vi "observacao.vi"() -> ()   [LabVIEW 2012] (continued)
                    n664 = global write "Global_Telescopio.vi" "T cup"(w581) -> ()
                    "Dome on Target" <- TRUE
                  }
                  frame True {
                    # "Abrir Trapeira"
                    n665 = case shown="False" w585 {
                      tunnel: [7 w590] -> w584
                      frame False {
                        w589 = u16 4 items=["ZERO", "AH", "DEC", "TUBO", "CUP"] ("Controlador")
                        # "Aguardar abertura Trap."
                        # "CLP Pronto"
                        n666 = call "Monta Comando.vi"("Comando"="ABRIR", "Dispositivo"="TRAPEIRA" ("Comando"), "Controlador"=w589) -> ()  [unwired: 4 in, 3 out]
                      }
                      frame True {
                        # "CLP Busy"
                        n667 = local read "TimeoutCUP"() -> (w592:u32)
                        n668 = call "TickTimeout.vi"("msInicial"=w592, "msTimeout"=u32 5000) -> ("Timeout"=w591:bool)  [unwired: 2 out]
                        n669 = case shown="True" w591 {
                          tunnel: [6 3] -> w590
                          frame False {
                          }
                          frame True {
                          }
                        }
                      }
                    }
                  }
                }
              }
              frame 7 {
                w596 = u16 6 items=["Alarme", "Atencao", "Erro", "Ocupado", "TBD", "LCB", "Trapeira", "Paravento", "DomoRap", "DomoCW", "DomoCCW", "TBD", "Em movimento", "TBD"] ("NomeStatus")
                # "Aqui também caberia um Timeout?"
                # "Aguarda abertura Trapeira"
                # "Também poderia ser testado o bit \"Em movimento\".\nNeste caso o código do \"IF\" deve ser permutado."
                n670 = call "Bit Status CUP.vi"("NomeStatus"=w596) -> ("StatBit"=w597:bool)
                n671 = case shown="True" w597 {
                  tunnel: [7 0] -> w598
                  frame False {
                    # "Ainda movendo...\nAGUARDAR"
                  }
                  frame True {
                    w601 = TRUE ("Dome on Target")
                    # "Trapeira aberta.\nFIM"
                    n672 = call "TickTimeout.vi"() -> ("msTick"=w600:u32)  [unwired: 2 in, 2 out]
                    n673 = local write "Dome on Target"(w601) -> ()
                    n674 = local write "RefreshShutterState"(w601) -> ()
                    n675 = local write "TimeoutCUP"(w600) -> ()
                    n676 = global write "Global_Telescopio.vi" "T cup"(w600) -> ()
                  }
                }
              }
            }
            n677 = case shown="True" w460 {
              tunnel: w449 -> [w480 _]
              tunnel: [w479 "POINT" ("Boolean Text.Text")] -> w448
              frame False {
                n678 = case shown="True" w480 {
                  tunnel: ["POINT" ("Boolean Text.Text") "STOP" ("Boolean Text.Text")] -> w479
                  frame False {
                  }
                  frame True {
                  }
                }
              }
              frame True {
                w483 = TRUE
                # "MUDANÇA:\n22/6/2011 \nHab. Guider"
                n679 = local read "ChkDomeEnable"() -> (w484:bool)
                n680 = global write "Global_Telescopio.vi" "Botão GO = STOP"(FALSE) -> ()
                n681 = local write "LED GUIDER"(w483) -> ()
                n682 = local write "GUIDER"(w483) -> ()
                n683 = local write "DOME"(w484) -> ()
              }
            }
            n684 = Tick Count (ms)() -> (millisecond timer value=w441:u32)
            n685 = Subtract(x=w441, y=w447) -> (x-y=w440:u32)
            n686 = Less?(x=w440, y=w442) -> (x < y?=w443:bool)
            n687 = control-ref of="BtTargetPoint"() -> (w477:refnum<vi>)
            n688 = case shown="True" w443 {
              tunnel: w442 -> [_ w478]
              frame False {
              }
              frame True {
                n689 = Wait Until Next ms Multiple(millisecond multiple=w478) -> ()  [unwired: 1 out]
              }
            }
            n690 = property class="Bool"(reference=w477, "Boolean Text.Text"=w448) -> ()  [unwired: 1 in, 2 out]
            n691 = call "PROTECAO.vi"("Estado In"=w453) -> ("Estado Out"=w452:i32)  [unwired: 2 in]
            n692 = local write "statCUP"(w452) -> ()
            "statCUP 2" <- "statCUP"
            "Erro Lim" <- 15 ("y")
            "Erro PROTEC" <- 10 ("y")
          }
          frame #4 {
            # "CHECA FINAL DO APONTAMENTO"
            # "ascensão reta = tempo sideral - ângulo horário (2)"
            n693 = local read "LedPointing"() -> (w899:bool)
            n694 = case shown="True" w899 {
              frame False {
                n695 = property on="DOME" class="Bool (strict)"("Disabled"=u8 0) -> ()  [unwired: 2 in, 2 out]
              }
              frame True {
                n696 = local read "statCUP"() -> (w904:i32)
                n697 = local read "statAH"() -> (w903:i32)
                n698 = local read "statDEC"() -> (w905:i32)
                n699 = Compound Arithmetic op=ADD(w904, w903, w905) -> (w906:i32)
                n700 = Greater Than 0?(x=w906) -> (x > 0?=w902:bool)
                n701 = case shown="False" w902 {
                  selector: w902 -> [w907 _]
                  frame False {
                    w910 = TRUE
                    n702 = local read "ChkPointPrecessed"() -> (w908:bool)
                    n703 = local read "StrPointObjName"() -> (w913:string)
                    n704 = local read "StrPointObjRA"() -> (w912:string)
                    n705 = local read "StrPointObjDEC"() -> (w911:string)
                    n706 = local write "LedPointing"(w907) -> ()
                    n707 = property on="LedPointing" class="Bool (strict)"("Visible"=w907) -> ()  [unwired: 2 in, 2 out]
                    n708 = case shown="True" w908 {
                      tunnel: ["2000.0" ("Saída") w915] -> w909
                      frame False {
                      }
                      frame True {
                        n709 = call "Calcula epoch.vi"() -> ("epoch"=w918:dbl)  [unwired: 2 in]
                        n710 = Number To Fractional String(number=w918, precision (6)=i16 1) -> (F-format string=w916:string)  [unwired: 2 in]
                        n711 = call "Comma_to_Point.vi"("Lat_A"=w916) -> ("Saída"=w915:string)
                      }
                    }
                    n712 = global write "Global_Telescopio.vi" "NAME OBJETO"(w913) -> ()
                    n713 = global write "Global_Telescopio.vi" "DEC AQUIS"(w911) -> ()
                    n714 = global write "Global_Telescopio.vi" "RA AQUIS"(w912) -> ()
                    n715 = local write "Processa Centragem"(w910) -> ()
                    n716 = property on="LedPointWorkArea" class="Bool (strict)"("Visible"=w910) -> ()  [unwired: 2 in, 2 out]
                    n717 = global write "Global_Telescopio.vi" "EPOCH AQUIS"(w909) -> ()
                  }
                  frame True {
                  }
                }
              }
            }
            n718 = local read "VARIABLE \nTRACKING"() -> (w900:bool)
            n719 = case shown="False" w900 {
              frame False {
              }
              frame True {
                n720 = local write "DEC"("DECTARGET") -> ()
                n721 = local write "RA"("AHTARGET") -> ()
              }
            }
          }
          frame #5 {
            # "PROCESSO OBJETO CENTRADO"
            n722 = case shown="True" "Processa Centragem" {
              frame False {
              }
              frame True {
                w927 = u16 3 items=["Alarme", "Atencao", "Erro", "Ocupado", "Protecao", "Embreagem", "Tracking", "Var. Track", "Rápido", "Ligeiro", "Médio", "Lento", "Em movimento", ""] ("NomeStatus")
                w928 = u16 3 items=["Alarme", "Atencao", "Erro", "Ocupado", "Protecao", "Embreagem", "Tracking", "Var. Track", "Rápido", "Ligeiro", "Médio", "Lento", "Em movimento", ""] ("NomeStatus")
                # "Roda case interno quando \nos controladores AH e DEC\nestiverem desocupados."
                n723 = call "Bit Status AH.vi"("NomeStatus"=w928) -> ("StatBit"=w926:bool)
                n724 = call "Bit Status DEC.vi"("NomeStatus"=w927) -> ("StatBit"=w925:bool)
                n725 = Or(x=w926, y=w925) -> (x .or. y?=w922:bool)
                n726 = case shown="False" w922 {
                  selector: w922 -> [w947 _]
                  tunnel: "INDEXER" ("Comando") -> [w949 _]
                  tunnel: "ZERAR" ("Comando") -> [w948 _]
                  frame False {
                    w935 = u16 1 items=["ZERO", "AH", "DEC", "TUBO", "CUP"] ("Controlador")
                    w936 = u16 2 items=["ZERO", "AH", "DEC", "TUBO", "CUP"] ("Controlador")
                    w929 = 0.0 ("AcumAG DEC")
                    # "PROCESSOPRECESSÃO"
                    # "PROCESSO ZERA POS_MOTOR"
                    # "Precessão"
                    n727 = local read "PM_RA"() -> (w941:string)
                    n728 = local read "Temp amb"() -> (w944:string)
                    n729 = local read "hum local"() -> (w942:string)
                    n730 = local read "MeanDEC"() -> (w945:string)
                    n731 = local read "pressão atm"() -> (w943:string)
                    n732 = local read "MeanRA"() -> (w946:string)
                    n733 = local read "PM_DEC"() -> (w940:string)
                    n734 = call "Monta Comando.vi"("Comando"=w948, "Dispositivo"=w949, "Controlador"=w935) -> ()  [unwired: 4 in, 3 out]
                    n735 = call "Monta Comando.vi"("Comando"=w948, "Dispositivo"=w949, "Controlador"=w936) -> ()  [unwired: 4 in, 3 out]
                    n736 = call "PrecessFortran.vi"("Asc reta"=w946, "Var RA"=w941, "Declinação"=w945, "Temperatura (Kelvin)"=w944, "Pressao atmosferica (mB)"=w943, "Humidade relativa (0 a 1)"=w942, "Var DEC"=w940) -> ("Observed RA (radians)"=w939:dbl, "Observed Dec (radians)"=w938:dbl)  [unwired: 2 in, 5 out]
                    n737 = local write "Processa Centragem"(w947) -> ()
                    n738 = global write "Global_Telescopio.vi" "LatchPrecRA"(w939) -> ()
                    n739 = global write "Global_Telescopio.vi" "LatchPrecDEC"(w938) -> ()
                    n740 = global read "Global_Telescopio.vi" "Sideral Time"() -> (w932:dbl)
                    n741 = global read "Global_Telescopio.vi" "PosDEC"() -> (w934:dbl)
                    n742 = global read "Global_Telescopio.vi" "PosAH"() -> (w933:dbl)
                    n743 = Subtract(x=w932, y=w933) -> (x-y=w931:dbl)
                    n744 = local write "LatchDeslocDEC"(w934) -> ()
                    n745 = local write "LatchDeslocRA"(w931) -> ()
                    n746 = global write "Global_Telescopio.vi" "AcumPrecDEC"(w929) -> ()
                    n747 = global write "Global_Telescopio.vi" "LatchAG RA"(w929) -> ()
                    n748 = global write "Global_Telescopio.vi" "AcumAG DEC"(w929) -> ()
                    n749 = global write "Global_Telescopio.vi" "AcumPrecRA"(w929) -> ()
                    n750 = global write "Global_Telescopio.vi" "LatchAG DEC"(w929) -> ()
                    n751 = global write "Global_Telescopio.vi" "AcumAG RA"(w929) -> ()
                    n752 = global write "Global_Telescopio.vi" "ObjCentrado"(TRUE) -> ()
                    n753 = property on="Calagem" class="Bool"("Disabled"=u8 0) -> ()  [unwired: 2 in, 2 out]
                  }
                  frame True {
                  }
                }
              }
            }
          }
          frame #6 {
            w953 = u16 2 items=["Alarme", "Atencao", "Erro", "Ocupado", "TBD", "LCB", "Trapeira", "Paravento", "DomoRap", "DomoCW", "DomoCCW", "TBD", "Em movimento", "TBD"] ("NomeStatus")
            w954 = u16 3 items=["Alarme", "Atencao", "Erro", "Ocupado", "TBD", "LCB", "Trapeira", "Paravento", "DomoRap", "DomoCW", "DomoCCW", "TBD", "Em movimento", "TBD"] ("NomeStatus")
            w958 = u16 3 items=["Alarme", "Atencao", "Erro", "Ocupado", "Protecao", "Embreagem", "Tracking", "Var. Track", "Rápido", "Ligeiro", "Médio", "Lento", "Em movimento", ""] ("NomeStatus")
            w959 = u16 3 items=["Alarme", "Atencao", "Erro", "Ocupado", "Protecao", "Embreagem", "Tracking", "Var. Track", "Rápido", "Ligeiro", "Médio", "Lento", "Em movimento", ""] ("NomeStatus")
            w967 = "ERROS" ("Comando")
            w970 = u16 2 items=["Alarme", "Atencao", "Erro", "Ocupado", "Protecao", "Embreagem", "Tracking", "Var. Track", "Rápido", "Ligeiro", "Médio", "Lento", "Em movimento", ""] ("NomeStatus")
            w971 = u16 2 items=["Alarme", "Atencao", "Erro", "Ocupado", "Protecao", "Embreagem", "Tracking", "Var. Track", "Rápido", "Ligeiro", "Médio", "Lento", "Em movimento", ""] ("NomeStatus")
            w968 = "PROG" ("Comando")
            # "LOGTCS ERROS"
            n754 = call "Bit Status AH.vi"("NomeStatus"=w971) -> ("StatBit"=w961:bool)
            n755 = call "Bit Status AH.vi"("NomeStatus"=w959) -> ("StatBit"=w957:bool)
            n756 = call "Bit Status DEC.vi"("NomeStatus"=w970) -> ("StatBit"=w960:bool)
            n757 = call "Bit Status DEC.vi"("NomeStatus"=w958) -> ("StatBit"=w956:bool)
            n758 = call "Bit Status CUP.vi"("NomeStatus"=w953) -> ("StatBit"=w969:bool)
            n759 = call "Bit Status CUP.vi"("NomeStatus"=w954) -> ("StatBit"=w966:bool)
            n760 = Not(x=w966) -> (.not. x?=w965:bool)
            n761 = Not(x=w957) -> (.not. x?=w963:bool)
            n762 = Not(x=w956) -> (.not. x?=w964:bool)
            n763 = And(x=w969, y=w965) -> (x .and. y?=w952:bool)
            n764 = And(x=w961, y=w963) -> (x .and. y?=w962:bool)
            n765 = And(x=w960, y=w964) -> (x .and. y?=w955:bool)
            n766 = And(x=FALSE, y=w952) -> (x .and. y?=w951:bool)
            n767 = case shown="True" w955 {
              selector: w955 -> [_ w980]
              tunnel: w968 -> [_ w981]
              tunnel: w967 -> [_ w977]
              frame False {
              }
              frame True {
                w978 = u16 2 items=["ZERO", "AH", "DEC", "TUBO", "CUP"] ("Controlador")
                n768 = call "Monta Comando.vi"("Comando"=w977, "Dispositivo"=w981, "Controlador"=w978) -> ("Resposta"=w979:string)  [unwired: 4 in, 2 out]
                n769 = call "Envia LOG.vi"("Error message"=w979, "Controlador"=w978, "Log de erro"=w980) -> ()  [unwired: 5 in, 2 out]
              }
            }
            n770 = case shown="True" w951 {
              selector: w951 -> [_ w975]
              tunnel: w968 -> [_ w976]
              tunnel: w967 -> [_ w972]
              frame False {
              }
              frame True {
                w973 = u16 4 items=["ZERO", "AH", "DEC", "TUBO", "CUP"] ("Controlador")
                n771 = call "Monta Comando.vi"("Comando"=w972, "Dispositivo"=w976, "Controlador"=w973) -> ("Resposta"=w974:string)  [unwired: 4 in, 2 out]
                n772 = call "Envia LOG.vi"("Error message"=w974, "Controlador"=w973, "Log de erro"=w975) -> ()  [unwired: 5 in, 2 out]
              }
            }
            n773 = case shown="True" w962 {
              selector: w962 -> [_ w985]
              tunnel: w968 -> [_ w986]
              tunnel: w967 -> [_ w982]
              frame False {
              }
              frame True {
                w983 = u16 1 items=["ZERO", "AH", "DEC", "TUBO", "CUP"] ("Controlador")
                n774 = call "Monta Comando.vi"("Comando"=w982, "Dispositivo"=w986, "Controlador"=w983) -> ("Resposta"=w984:string)  [unwired: 4 in, 2 out]
                n775 = call "Envia LOG.vi"("Error message"=w984, "Controlador"=w983, "Log de erro"=w985) -> ()  [unwired: 5 in, 2 out]
              }
            }
          }
          frame #7 {
            # "MASSA DE AR"
            # "z'"
            # "z * (1 - 0,0012* (z* z -1) )"
            # "(z* z -1)"
            # "z"
            # "O Hour Angle é calculado com essa equação (AH = TS - RA), \nsendo TS o tempo sideral que você fica calculando o tempo todo e RA a \ncoordenada que vem do quadro TARGET da aba POINTING."
            # "Coslat"
            # "Sinlat"
            # "MASSA DE AR\n# define LAT -22,534444444444 / / Lat itude do telescópio\n# define SINLAT -0,383238771 / / Seno da Lat itude\n# define COSLAT 0,923649308 / / Cosseno da Lat itude\ndouble airmass (double ah, double delta) / / ângulos dos eixos AH e DEC em radianos\n{ double z;\nz = 1./ (SINLAT* sin(delta) + COSLAT* cos(delta) * cos(ah) ) ;\nz = z * (1 - 0,0012* (z* z -1) ) ;\nif (z > = 10) z = 9.999;\nif (z < 0) z = 0;\nreturn (z) ;\n}"
            n776 = global read "Global_Telescopio.vi" "AH_now"() -> (w987:dbl)
            n777 = global read "Global_Telescopio.vi" "delta_now"() -> (w988:dbl)
            n778 = Cosine(x=w988) -> (cos(x)=w1008:dbl)
            n779 = Sine(x=w988) -> (sin(x)=w1010:dbl)
            n780 = Cosine(x=w987) -> (cos(x)=w1006:dbl)
            n781 = Multiply(x=0.923649308 ("Delta=DEC"), y=w1008) -> (x*y=w1007:dbl)
            n782 = Multiply(x=-0.383238771 ("Delta=DEC"), y=w1010) -> (x*y=w1005:dbl)
            n783 = Multiply(x=w1007, y=w1006) -> (x*y=w1004:dbl)
            n784 = Add(x=w1005, y=w1004) -> (x+y=w1003:dbl)
            n785 = Reciprocal(x=w1003) -> (1/x=w995:dbl)
            n786 = Subtract(x=w995, y=1.0) -> (x-y=w1001:dbl)
            n787 = Multiply(x=w995, y=w1001) -> (x*y=w1000:dbl)
            n788 = Multiply(x=w1000, y=0.0012) -> (x*y=w997:dbl)
            n789 = Subtract(x=1.0 ("y"), y=w997) -> (x-y=w996:dbl)
            n790 = Multiply(x=w995, y=w996) -> (x*y=w992:dbl)
            n791 = Greater Or Equal?(x=w992, y=10.0) -> (x >= y?=w993:bool)
            n792 = case shown="True" w993 {
              tunnel: [w1014 9.999999 ("y")] -> w990
              tunnel: w992 -> [w1014 _]
              frame False {
              }
              frame True {
              }
            }
            n793 = Less Than 0?(x=w990) -> (x < 0?=w991:bool)
            n794 = case shown="True" w991 {
              tunnel: [w1012 0.0 ("y")] -> w989
              tunnel: w990 -> [w1012 _]
              frame False {
              }
              frame True {
              }
            }
            "Air Mass" <- w989
            n795 = global write "Global_Telescopio.vi" "Air Mass"(w989) -> ()
          }
          frame #8 {
          }
          frame #9 {
            # "CONDIÇÕES ATMOSFÉRICAS"
            # "Se mudou a Chave\ngera um Pulso"
            # "A cada n Segundos\nEssa rotina gera 1\npulso!"
            # "Seg"
            # "Janela Das Condições Atmosféricas"
            n796 = local read "Int/Ext"() -> (w1018:bool)
            n797 = global read "Global_Telescopio.vi" "Default Met"() -> (w1016:bool)
            n798 = call "timepulse.vi"("de quantos segundos"=i16 10) -> ("PULSO"=w1022:bool)  [unwired: 2 in]
            n799 = call "Pulso_se_Mudou.vi"("Entrada"=w1018) -> ("Saída"=w1019:bool)
            n800 = local write "Default Met"(w1016) -> ()
            n801 = Or(x=w1019, y=w1022) -> (x .or. y?=w1020:bool)
            n802 = case shown="True" w1020 {
              tunnel: [_ TRUE ("Int/Ext")] -> w1017
              frame False {
              }
              frame True {
                n803 = stacked-sequence {
                  frame #0 {
                    # "O botão INT/ EXT (cf. figura 3) seleciona se os most radores TEMPERATURE, HUMIDITY\ne DEW POINT são atualizados com os valores internos ou externos desse regist ro.\nA barra gráfica CLOUSURE LIMITS deve ser deslocada em função da proximidade\n(dada por um valor percentural de zero a 100%) dos valores lidos do arquivo de dados\natmosféricos com os valores- limite das grandezas listadas nesse quadro. Para\nPRESSURE e WIND SPEED, considerar os valores- limite desse quadro como o final de\numa escala de 0 a 100%, cujo valor inicial (0%) corresponde ao valor zero dessas\ngrandezas. Para as grandezas DEWPOINT, interna e externa, considerar os valores\nlimites listados no quadro como final da escala (100%) e cada décimo de ºC acima\ndos valores- limite como 1% da escala."
                    # "A simulação da janela ENVIRONMENT STATUS será feita com os dados de um arquivo\ngerado pela estação meteorológica contendo os regist ros de 24 horas de monitoria,\nsendo cada regist ro efetuado em intervalos de 10 minutos. A simulação deve procurar\nnesse arquivo (anexo, LNA-TCSPD-MP-00012-01-100.txt ) o regist ro correspondente à\nhora local do PC, ler esse regist ro e ret irar as informações de cada most rador para\natualizar essa janela."
                  }
                  frame #1 {
                    w1034 = "\t"
                    (unwired) "1:04" ("Hora a ser Procurada")
                    # "Lê arquivo, da Est. Meteor."
                    # "MUDANÇA FUTURA:\nSe possível, mostrar os valores de Pressão atm,\nTemp. amb. e umidade rel.\nda estação do tubo em lugar\ndos valores internos."
                    # "O Fortran usa valores\nde umidade entre 0 e 1."
                    # "MUDANÇA 08/04/2011:\nCriada a variável AtmosferaStr para guardar dados\nmeteorológicos para Erros de Apontamento"
                    # "Celsius -->Kelvin\nO Fortran usa Kelvin"
                    # "bar"
                    # "Formato"
                    n804 = case shown="False" "Default Met" {
                      tunnel: ["OFF" "ON"] -> w1032
                      frame False {
                      }
                      frame True {
                      }
                    }
                    n805 = case shown="False" "Int/Ext" {
                      tunnel: [27 ("index") 2 ("index")] -> w1066
                      tunnel: [28 ("index") 5 ("index")] -> w1065
                      tunnel: [29 ("index") 6 ("index")] -> w1064
                      frame False {
                        # "Interno"
                      }
                      frame True {
                        # "Externo"
                      }
                    }
                    n806 = property on="Default" class="Str"("Visible"="Default Met") -> ()  [unwired: 2 in, 2 out]
                    n807 = global write "Global_Telescopio.vi" "WS_DEFAULT"(w1032) -> ()
                    n808 = case shown="False" "Default Met" {
                      tunnel: [w1093 string[] ["24/05/18", "13:00", "19.1", "19.1", "19.1", "61", "11.4", "2.2", "NNW", "0.67", "4.5", "NNW", "19.1", "18.8", "18.8", "24.1", "761.5", "0.00", "0.0", "705", "5.05", "710", "5.9", "0.21", "5.9", "0.000", "0.003", "17.6", "53", "7.9", "16.7", "20.6", "16.7", "40", "50", "0.43", "0", "113", "1", "99.1", "5", "\r\n", "", "", "", "", ""] ("Array")] -> w1089
                      frame False {
                        n809 = call "Procura_no_Arquivo.vi"() -> ("Erro de Leitura=True"=w1092:bool, "Array"=w1093:string[])  [unwired: 4 in]
                        n810 = local write "Default Met"(w1092) -> ()
                      }
                      frame True {
                      }
                    }
                    n811 = Index Array(array=w1089, index #1=w1066, index #2=w1065, index #3=w1064, index #4=7 ("index"), index #5=8 ("index"), index #6=12 ("index"), index #7=16 ("index"), index #8=2 ("index"), index #9=5 ("index"), index #10=27 ("index"), index #11=28 ("index"), index #12=36 ("index")) -> (element #1=w1075:string, element #2=w1088:string, element #3=w1085:string, element #4=w1081:string, element #5=w1035:string, element #6=w1080:string, element #7=w1076:string, element #8=w1049:string, element #9=w1048:string, element #10=w1045:string, element #11=w1044:string, element #12=w1026:string)
                    "Wind Dir" <- w1035
                    n812 = Decimal String To Number(string=w1026) -> (number=→"LEAF":i32)  [unwired: 2 in, 1 out]
                    n813 = call "point_to_comma.vi"("Lat_A"=w1075) -> ("Saída"=w1071:string)
                    n814 = call "point_to_comma.vi"("Lat_A"=w1088) -> ("Saída"=w1072:string)
                    n815 = call "point_to_comma.vi"("Lat_A"=w1085) -> ("Saída"=w1038:string)
                    n816 = call "point_to_comma.vi"("Lat_A"=w1081) -> ("Saída"=w1036:string)
                    n817 = call "point_to_comma.vi"("Lat_A"=w1080) -> ("Saída"=w1037:string)
                    n818 = call "point_to_comma.vi"("Lat_A"=w1076) -> ("Saída"=w1041:string)
                    "pressão atm" <- w1041
                    n819 = call "point_to_comma.vi"("Lat_A"=w1049) -> ("Saída"=w1043:string)
                    n820 = call "point_to_comma.vi"("Lat_A"=w1048) -> ("Saída"=w1042:string)
                    n821 = call "point_to_comma.vi"("Lat_A"=w1045) -> ("Saída"=w1040:string)
                    n822 = call "point_to_comma.vi"("Lat_A"=w1044) -> ("Saída"=w1039:string)
                    n823 = Concatenate Strings(w1043, w1034, w1042, w1034, w1041, w1034, w1040, w1034, w1039, w1034, w1038, w1034, w1036, w1034, w1035, w1034) -> (→"AtmosferaStr":string)
                    n824 = Fract/Exp String To Number(string=w1071, default (0 dbl)=1.0 ("default (0 DBL)")) -> (number=w1031:dbl)  [unwired: 2 in, 1 out]
                    "Temperature" <- w1031
                    n825 = Fract/Exp String To Number(string=w1072, default (0 dbl)=1.0 ("default (0 DBL)")) -> (number=w1030:dbl)  [unwired: 2 in, 1 out]
                    "Humidity" <- w1030
                    n826 = Fract/Exp String To Number(string=w1038, default (0 dbl)=1.0 ("default (0 DBL)")) -> (number=→"Dew Point":dbl)  [unwired: 2 in, 1 out]
                    n827 = Fract/Exp String To Number(string=w1036, default (0 dbl)=1.0 ("default (0 DBL)")) -> (number=→"Wind Speed":dbl)  [unwired: 2 in, 1 out]
                    n828 = Fract/Exp String To Number(string=w1037, default (0 dbl)=1.0 ("default (0 DBL)")) -> (number=→"Wind Chill":dbl)  [unwired: 2 in, 1 out]
                    n829 = Fract/Exp String To Number(string=w1041, default (0 dbl)=1.0 ("default (0 DBL)")) -> (number=w1029:dbl)  [unwired: 2 in, 1 out]
                    "Pressure" <- w1029
                    n830 = Fract/Exp String To Number(string=w1043, default (0 dbl)=1.0 ("default (0 DBL)")) -> (number=w1052:dbl)  [unwired: 2 in, 1 out]
                    n831 = Fract/Exp String To Number(string=w1042, default (0 dbl)=1.0 ("default (0 DBL)")) -> (number=w1051:dbl)  [unwired: 2 in, 1 out]
                    n832 = Add(x=w1052, y=273.5 ("default (0 DBL)")) -> (x+y=w1069:dbl)
                    n833 = Divide(x=w1051, y=100.0 ("default (0 DBL)")) -> (x/y=w1054:dbl)
                    n834 = global write "Global_Telescopio.vi" "BAR"(w1029) -> ()
                    n835 = global write "Global_Telescopio.vi" "HUM"(w1030) -> ()
                    n836 = global write "Global_Telescopio.vi" "TEMP"(w1031) -> ()
                    n837 = Number To Fractional String(number=w1069, precision (6)=i16 1) -> (F-format string=→"Temp amb":string)  [unwired: 2 in]
                    n838 = Number To Fractional String(number=w1054, precision (6)=i16 2) -> (F-format string=→"hum local":string)  [unwired: 2 in]
                  }
                  frame #2 {
                    # "Em relação as suas perguntas:\n- Temperaturas (Temperature, Dew Point e Wind Chill): mínimo/máximo: -20 a +50 graus\n- Humidity:  0 a 100%\n- Pressão atmosférica: de 300 a 1200 mBar\n- Velocidade do vento: 0 a 300 Km/h\n\nNotar que a chave INT/EXT na parte superior do quadro \nesquerdo seleciona se são mostrados os valores internos ou externos de Temperatura, Umidade e Dew Point."
                    # "Pressure Max"
                    # "Wind chill Point Max"
                    # "Temp Point Max"
                    # "Dew Point Max"
                    # "Humidity Max"
                    # "Speed Max"
                    # "Steady Wind           >  70 Km/h\nRelative Humidity    >  97 %\nInternal Dewpoint  <  0.5  C\nExternal Dewpoint <  1.0  C"
                    n839 = Divide(x=100.0, y=300.0 ("x")) -> (x/y=w1132:dbl)
                    n840 = local read "Wind Speed"() -> (w1131:dbl)
                    n841 = Divide(x=100.0, y=100.0 ("x")) -> (x/y=w1126:dbl)
                    n842 = local read "Humidity"() -> (w1125:dbl)
                    n843 = local read "Dew Point"() -> (w1121:dbl)
                    n844 = Divide(x=100.0, y=50.0 ("x")) -> (x/y=w1118:dbl)
                    n845 = Divide(x=100.0, y=1200.0 ("x")) -> (x/y=w1112:dbl)
                    n846 = Divide(x=100.0, y=50.0 ("x")) -> (x/y=w1124:dbl)
                    n847 = Divide(x=100.0, y=50.0 ("x")) -> (x/y=w1117:dbl)
                    n848 = Multiply(x=w1131, y=w1132) -> (x*y=w1108:dbl)
                    n849 = local read "Temperature"() -> (w1109:dbl)
                    n850 = local read "Wind Chill"() -> (w1110:dbl)
                    n851 = local read "Pressure"() -> (w1111:dbl)
                    n852 = Multiply(x=w1125, y=w1126) -> (x*y=w1107:dbl)
                    n853 = Multiply(x=w1109, y=w1118) -> (x*y=w1105:dbl)
                    n854 = Multiply(x=w1111, y=w1112) -> (x*y=w1103:dbl)
                    n855 = Multiply(x=w1121, y=w1124) -> (x*y=w1106:dbl)
                    n856 = Multiply(x=w1110, y=w1117) -> (x*y=w1104:dbl)
                    n857 = Build Array(w1108, w1107, w1106, w1105, w1104, w1103) -> (w1102:dbl[])
                    n858 = Array Max & Min(array=w1102) -> (max value=w1101:dbl)  [unwired: 3 out]
                    n859 = local write "SlideEnviromental"(w1101) -> ()
                  }
                  frame #3 {
                    # "Determinadas as proximidades de cada grandeza em valores percentuais, selecionar o\nvalor da mais elevada para ser most rado na barra gráfica. A cor dessa barra gráfica\ndeve mudar em função do valor most rado. Enquanto est iver abaixo de 90%, ela deve\nser verde, ent re 90 e 95% amarela e acima de 95% vermelha. O led ao lado desse\nbarra deve ficar ligado e ter a mesma cor da barra gráfica, mas quando esta\nult rapassar 90%, ou seja quando for amarela ou vermelha, o led deve piscar."
                    n860 = local read "SlideEnviromental"() -> (w1133:dbl)
                    n861 = In Range and Coerce(upper limit=95.0 ("lower limit"), x=w1133, lower limit=90.0 ("upper limit")) -> (In Range?=w1138:bool)  [unwired: 1 out]
                    n862 = Less?(x=w1133, y=90.0) -> (x < y?=w1140:bool)
                    n863 = Greater?(x=w1133, y=95.0 ("lower limit")) -> (0:w1137:bool)
                    n864 = case shown="True" w1138 {
                      frame False {
                      }
                      frame True {
                        n865 = stacked-sequence {
                          frame #0 {
                            n866 = property on="SlideEnviromental" class="Slide (strict)"("Fill Color"=u32 16772882) -> ()  [unwired: 2 in, 2 out]
                            n867 = local write "Boolean 11"(TRUE ("Boolean 11")) -> ()
                            n868 = property on="Boolean 11" class="Bool (strict)"("Blinking"=FALSE) -> ()  [unwired: 2 in, 2 out]
                          }
                          frame #1 {
                            # "Cor do Led"
                            # "lig"
                            # "des"
                            n869 = Bundle(u32 7171459, u32 46096) -> (w1160:cluster{u32, u32})  [unwired: 1 in]
                            n870 = Bundle(u32 16772882, u32 46096) -> (w1159:cluster{u32, u32})  [unwired: 1 in]
                            n871 = Build Array(w1160, w1159) -> (w1158:cluster{u32, u32}[])
                            n872 = property on="Boolean 11" class="Bool (strict)"("Colors [4]"=w1158) -> ()  [unwired: 2 in, 2 out]
                          }
                        }
                      }
                    }
                    n873 = case shown="True" w1140 {
                      frame False {
                      }
                      frame True {
                        n874 = stacked-sequence {
                          frame #0 {
                            n875 = property on="SlideEnviromental" class="Slide (strict)"("Fill Color"=u32 6618880) -> ()  [unwired: 2 in, 2 out]
                            n876 = local write "Boolean 11"(TRUE ("Boolean 11")) -> ()
                            n877 = property on="Boolean 11" class="Bool (strict)"("Blinking"=FALSE) -> ()  [unwired: 2 in, 2 out]
                          }
                          frame #1 {
                            # "Cor do Led"
                            # "lig"
                            # "des"
                            n878 = Bundle(u32 7171459, u32 46096) -> (w1164:cluster{u32, u32})  [unwired: 1 in]
                            n879 = Bundle(u32 6618880, u32 46096) -> (w1165:cluster{u32, u32})  [unwired: 1 in]
                            n880 = Build Array(w1164, w1165) -> (w1166:cluster{u32, u32}[])
                            n881 = property on="Boolean 11" class="Bool (strict)"("Colors [4]"=w1166) -> ()  [unwired: 2 in, 2 out]
                          }
                        }
                      }
                    }
                    n882 = case shown="True" w1137 {
                      frame False {
                      }
                      frame True {
                        n883 = stacked-sequence {
                          frame #0 {
                            n884 = local write "Boolean 11"(TRUE ("Boolean 11")) -> ()
                            n885 = property on="SlideEnviromental" class="Slide (strict)"("Fill Color"=u32 16715776) -> ()  [unwired: 2 in, 2 out]
                            n886 = property on="Boolean 11" class="Bool (strict)"("Blinking"=TRUE) -> ()  [unwired: 2 in, 2 out]
                          }
                          frame #1 {
                            # "Cor do Led"
                            # "lig"
                            # "des"
                            n887 = Bundle(u32 7171459, u32 46096) -> (w1144:cluster{u32, u32})  [unwired: 1 in]
                            n888 = Bundle(u32 16715776, u32 46096) -> (w1145:cluster{u32, u32})  [unwired: 1 in]
                            n889 = Build Array(w1144, w1145) -> (w1146:cluster{u32, u32}[])
                            n890 = property on="Boolean 11" class="Bool (strict)"("Colors [4]"=w1146) -> ()  [unwired: 2 in, 2 out]
                          }
                        }
                      }
                    }
                  }
                }
              }
            }
            n891 = flat-sequence {
              tunnel: w1017 -> [_]
              frame #0 {
                n892 = local read "LEAF"() -> (w1023:i32)
                n893 = call "Testa_Leaf.vi"("LEAF"=w1023) -> ()  [unwired: 11 in]
              }
            }
          }
          frame #10 {
            w1181 = u16 3 items=["Alarme", "Atencao", "Erro", "Ocupado", "Protecao", "Embreagem", "Tracking", "Var. Track", "Rápido", "Ligeiro", "Médio", "Lento", "Em movimento", ""] ("NomeStatus")
            w1182 = u16 3 items=["Alarme", "Atencao", "Erro", "Ocupado", "Protecao", "Embreagem", "Tracking", "Var. Track", "Rápido", "Ligeiro", "Médio", "Lento", "Em movimento", ""] ("NomeStatus")
            # "PROCESSO AUTO GUIDER"
            n894 = local read "MOUNT"() -> (w1178:bool)
            n895 = local read "LedPointing"() -> (w1176:bool)
            n896 = global read "Global_Telescopio.vi" "Correção Guider"() -> (w1172:bool)
            n897 = local read "MOVING"() -> (w1175:bool)
            n898 = call "Bit Status AH.vi"("NomeStatus"=w1182) -> ("StatBit"=w1179:bool)
            n899 = call "Bit Status DEC.vi"("NomeStatus"=w1181) -> ("StatBit"=w1180:bool)
            n900 = Not(x=w1175) -> (.not. x?=w1174:bool)
            n901 = Not(x=w1176) -> (.not. x?=w1173:bool)
            n902 = Not Or(1:w1180, 2:w1179) -> (0:w1177:bool)
            n903 = Compound Arithmetic op=AND(w1172, w1173, w1174, "GUIDER", w1178, w1177) -> (w1183:bool)
            n904 = case shown="True" w1183 {
              frame False {
                # "Reseta Flag da comunicação do Guider"
                n905 = global write "Global_Telescopio.vi" "Correção Guider"(FALSE ("Correção Guider")) -> ()
              }
              frame True {
                # "MUDANÇA:\n(25/08/2010)"
                # "É necessário testar se as\nstrings são igual a espaço\nem virtude de um BUG,\nno Soft do Auto guider!"
                n906 = global read "Global_Telescopio.vi" "guide_dir_ns"() -> (w1190:string)
                n907 = global read "Global_Telescopio.vi" "guide_dir_we"() -> (w1191:string)
                n908 = case shown="\"W\"" w1191 {
                  tunnel: [0.0 ("PreciseOffsetDEC 2") 1.0 ("PreciseOffsetDEC 2") -1.0 ("PreciseOffsetDEC 2")] -> w1188
                  frame " ", Default {
                  }
                  frame "W" {
                  }
                  frame "E" {
                  }
                }
                n909 = case shown="\"N\"" w1190 {
                  tunnel: [0.0 ("PreciseOffsetDEC 2") 1.0 ("PreciseOffsetDEC 2") -1.0 ("PreciseOffsetDEC 2")] -> w1187
                  frame " ", Default {
                  }
                  frame "N" {
                  }
                  frame "S" {
                  }
                }
                n910 = Equal To 0?(x=w1188) -> (x = 0?=w1185:bool)
                n911 = Equal To 0?(x=w1187) -> (x = 0?=w1186:bool)
                n912 = And(x=w1185, y=w1186) -> (x .and. y?=w1189:bool)
                n913 = case shown="False" w1189 {
                  tunnel: w1188 -> [w1196 _]
                  tunnel: w1187 -> [w1195 _]
                  frame False {
                    # "Comandos do Auto guider contendo direção"
                    n914 = global read "Global_Telescopio.vi" "esc_placa"() -> (w1194:string)
                    n915 = Fract/Exp String To Number(use system decimal point (T)=FALSE, string=w1194) -> (number=w1193:dbl)  [unwired: 2 in, 1 out]
                    n916 = stacked-sequence {
                      tunnel: w1196 -> [w1202 _ _]
                      tunnel: w1195 -> [_ w1222 _]
                      tunnel: w1193 -> [w1199 w1219 _]
                      frame #0 {
                        n917 = local read "AtualDEC"() -> (w1207:dbl)
                        n918 = global read "Global_Telescopio.vi" "CorrecaoMin"() -> (w1197:dbl)
                        n919 = global read "Global_Telescopio.vi" "guide_asc"() -> (w1201:dbl)
                        n920 = Cosine(x=w1207) -> (cos(x)=w1206:dbl)
                        n921 = Multiply(x=w1201, y=w1199) -> (x*y=w1200:dbl)
                        n922 = Absolute Value(x=w1206) -> (abs(x)=w1205:dbl)
                        n923 = Divide(x=w1200, y=w1205) -> (x/y=w1203:dbl)
                        n924 = Multiply(x=w1202, y=w1203) -> (x*y=w1198:dbl)
                        n925 = Greater?(x=w1203, y=w1197) -> (0:w1204:bool)
                        n926 = case shown="True" w1204 {
                          tunnel: w1198 -> [_ w1209]
                          frame False {
                          }
                          frame True {
                            w1213 = u16 1 items=["ZERO", "AH", "DEC", "TUBO", "CUP"] ("Controlador")
                            # "PROCESSO MOVE TELESCÓPIO"
                            n927 = local read "Offset RA"() -> (w1210:dbl)
                            n928 = Add(x=w1209, y=w1210) -> (x+y=w1211:dbl)
                            n929 = property on="Calagem" class="Bool"("Disabled"=u8 2) -> ()  [unwired: 2 in, 2 out]
                            n930 = call "Conversao Ms to Hora texto.vi"("TRUE=HORA\nFALSE=GRAU"=TRUE ("TRUE=HORA\nFALSE=GRAU"), "PrecDEC"=w1209) -> ("Hora/Graus Texto Decimal"=w1216:string)
                            n931 = local write "Offset RA"(w1211) -> ()
                            n932 = call "Monta Comando.vi"("Set Point"=w1216, "Comando"="MOVER_REL", "Dispositivo"="EIXO" ("Comando"), "Controlador"=w1213) -> ()  [unwired: 3 in, 3 out]
                          }
                        }
                      }
                      frame #1 {
                        n933 = global read "Global_Telescopio.vi" "guide_dec"() -> (w1221:dbl)
                        n934 = Multiply(x=w1221, y=w1219) -> (x*y=w1220:dbl)
                        n935 = global read "Global_Telescopio.vi" "CorrecaoMin"() -> (w1217:dbl)
                        n936 = Greater?(x=w1220, y=w1217) -> (0:w1223:bool)
                        n937 = Multiply(x=w1222, y=w1220) -> (x*y=w1218:dbl)
                        n938 = case shown="True" w1223 {
                          tunnel: w1218 -> [_ w1225]
                          frame False {
                          }
                          frame True {
                            w1229 = u16 2 items=["ZERO", "AH", "DEC", "TUBO", "CUP"] ("Controlador")
                            # "PROCESSO MOVE TELESCÓPIO"
                            n939 = local read "Offset DEC"() -> (w1226:dbl)
                            n940 = Add(x=w1225, y=w1226) -> (x+y=w1227:dbl)
                            n941 = property on="Calagem" class="Bool"("Disabled"=u8 2) -> ()  [unwired: 2 in, 2 out]
                            n942 = call "Conversao Ms to Hora texto.vi"("TRUE=HORA\nFALSE=GRAU"=FALSE ("TRUE=HORA\nFALSE=GRAU"), "PrecDEC"=w1225) -> ("Hora/Graus Texto Decimal"=w1232:string)
                            n943 = local write "Offset DEC"(w1227) -> ()
                            n944 = call "Monta Comando.vi"("Set Point"=w1232, "Comando"="MOVER_REL", "Dispositivo"="EIXO" ("Comando"), "Controlador"=w1229) -> ()  [unwired: 3 in, 3 out]
                          }
                        }
                      }
                      frame #2 {
                        # "Reseta Flag da comunicação do Guider"
                        n945 = global write "Global_Telescopio.vi" "Correção Guider"(FALSE ("Correção Guider")) -> ()
                      }
                    }
                  }
                  frame True {
                  }
                }
              }
            }
            "LED GUIDER" <- "GUIDER"
          }
          frame #11 {
            w1249 = u16 12 items=["Alarme", "Atencao", "Erro", "Ocupado", "Protecao", "Embreagem", "Tracking", "Var. Track", "Rápido", "Ligeiro", "Médio", "Lento", "Em movimento", ""] ("NomeStatus")
            w1248 = u16 12 items=["Alarme", "Atencao", "Erro", "Ocupado", "Protecao", "Embreagem", "Tracking", "Var. Track", "Rápido", "Ligeiro", "Médio", "Lento", "Em movimento", ""] ("NomeStatus")
            # "Aqui era a Global\nLIMITE"
            # "Este teste deve ser executado antes do Frame de enviar\ncomando do sistema de aquisição, em virtude de teste do \nmovimento."
            # "Quando o Movimento Parar\nreseta a Variável/Flag para enviar \no CR ao sitema de Aquisição"
            n946 = global read "Global_Telescopio.vi" "AQ Offset Mov"() -> (w1245:bool)
            n947 = call "Bit Status AH.vi"("NomeStatus"=w1248) -> ("StatBit"=w1251:bool)
            n948 = call "Bit Status DEC.vi"("NomeStatus"=w1249) -> ("StatBit"=w1250:bool)
            n949 = local read "Proteção"() -> (w1241:bool)
            n950 = Not Or(1:w1250, 2:w1251) -> (0:w1246:bool)
            n951 = case shown="True" w1241 {
              selector: w1241 -> [w1252 w1253]
              frame False {
                n952 = local write "LIMITE"(w1252) -> ()
                n953 = property on="LIMITE" class="Bool"("Blinking"=w1252) -> ()  [unwired: 2 in, 2 out]
              }
              frame True {
                n954 = property on="LIMITE" class="Bool"("Blinking"=w1253) -> ()  [unwired: 2 in, 2 out]
                "LIMITE" <- w1253
              }
            }
            n955 = And(x=w1245, y=w1246) -> (x .and. y?=w1247:bool)
            n956 = case shown="True" w1247 {
              frame False {
              }
              frame True {
                n957 = global write "Global_Telescopio.vi" "AQ Offset Mov"(FALSE ("AQ Offset Mov")) -> ()
              }
            }
            n958 = global read "Global_Telescopio.vi" "Z_SEGURANÇA_GRAUS"() -> (w1244:dbl)
            n959 = global read "Global_Telescopio.vi" "Zenital angle GRAUS"() -> (w1243:dbl)
            n960 = global read "Global_Telescopio.vi" "FinalsFileDownload"() -> (→"Precess Data out-of-date":bool)
            n961 = Greater?(x=w1243, y=w1244) -> (0:→"Security Zone":bool)
          }
          frame #12 {
            w1268 = u16 8 items=["Alarme", "Atencao", "Erro", "Ocupado", "Protecao", "Embreagem", "Tracking", "Var. Track", "Rápido", "Ligeiro", "Médio", "Lento", "Em movimento", ""] ("NomeStatus")
            w1269 = u16 8 items=["Alarme", "Atencao", "Erro", "Ocupado", "Protecao", "Embreagem", "Tracking", "Var. Track", "Rápido", "Ligeiro", "Médio", "Lento", "Em movimento", ""] ("NomeStatus")
            # "ATUALIZAÇÃO DO QUADRO STATUS INFORMATION"
            n962 = call "Bit Status DEC.vi"("NomeStatus"=w1268) -> ("StatBit"=w1266:bool)
            n963 = call "Bit Status AH.vi"("NomeStatus"=w1269) -> ("StatBit"=w1267:bool)
            n964 = global read "Global_Telescopio.vi" "Bit RX Aquis"() -> (w1261:bool)
            n965 = global read "Global_Telescopio.vi" "Bit RX Guider"() -> (w1262:bool)
            n966 = Or(x=w1267, y=w1266) -> (x .or. y?=w1265:bool)
            n967 = case shown="True" w1261 {
              selector: w1261 -> [w1278 w1280]
              frame False {
                n968 = local write "Data Acquisition Activity"(w1278) -> ()
              }
              frame True {
                # "Liga Led RX por 1 ciclo"
                n969 = global write "Global_Telescopio.vi" "Bit RX Aquis"(FALSE) -> ()
                "Data Acquisition Activity" <- w1280
              }
            }
            n970 = case shown="True" w1262 {
              selector: w1262 -> [w1281 w1282]
              frame False {
                n971 = local write "Auto guider Activity"(w1281) -> ()
              }
              frame True {
                # "Liga Led RX por 1 ciclo"
                n972 = global write "Global_Telescopio.vi" "Bit RX Guider"(FALSE) -> ()
                "Auto guider Activity" <- w1282
              }
            }
            n973 = case shown="False" w1265 {
              tunnel: [FALSE w1294] -> w1264
              tunnel: [w1284 w1295] -> w1263
              frame False {
                w1288 = u16 10 items=["Alarme", "Atencao", "Erro", "Ocupado", "Protecao", "Embreagem", "Tracking", "Var. Track", "Rápido", "Ligeiro", "Médio", "Lento", "Em movimento", ""] ("NomeStatus")
                w1287 = u16 10 items=["Alarme", "Atencao", "Erro", "Ocupado", "Protecao", "Embreagem", "Tracking", "Var. Track", "Rápido", "Ligeiro", "Médio", "Lento", "Em movimento", ""] ("NomeStatus")
                w1292 = u16 9 items=["Alarme", "Atencao", "Erro", "Ocupado", "Protecao", "Embreagem", "Tracking", "Var. Track", "Rápido", "Ligeiro", "Médio", "Lento", "Em movimento", ""] ("NomeStatus")
                w1293 = u16 9 items=["Alarme", "Atencao", "Erro", "Ocupado", "Protecao", "Embreagem", "Tracking", "Var. Track", "Rápido", "Ligeiro", "Médio", "Lento", "Em movimento", ""] ("NomeStatus")
                n974 = call "Bit Status AH.vi"("NomeStatus"=w1293) -> ("StatBit"=w1291:bool)
                n975 = call "Bit Status DEC.vi"("NomeStatus"=w1292) -> ("StatBit"=w1290:bool)
                n976 = call "Bit Status AH.vi"("NomeStatus"=w1287) -> ("StatBit"=w1286:bool)
                n977 = call "Bit Status DEC.vi"("NomeStatus"=w1288) -> ("StatBit"=w1285:bool)
                n978 = Compound Arithmetic op=OR(w1291, w1290, w1286, w1285) -> (w1284:bool)
              }
              frame True {
                w1294 = TRUE
                n979 = Not(x=w1294) -> (.not. x?=w1295:bool)
              }
            }
            "Mount Gross Movement" <- w1264
            "Mount Fine Movement" <- w1263
            n980 = case shown="True" "News" {
              selector: "News" -> [_ w1274]
              frame False {
              }
              frame True {
                n981 = flat-sequence {
                  tunnel: w1274 -> [w1275]
                  frame #0 {
                    n982 = call "Monta_Mensagem.vi"("Zerar"=w1275) -> ()  [unwired: 2 in]
                  }
                  frame #1 {
                    n983 = global write "Global_Telescopio.vi" "SYSTEM MESSAGES"("Na janela de SETUP->Configuracao, o endereco do arquivo \"finals2000A.all\" (usado para calculos de  precessao) passou a ser editavel." ("SYSTEM MESSAGES")) -> ()
                  }
                }
              }
            }
            n984 = global read "Global_Telescopio.vi" "SYSTEM MESSAGES"() -> (→"SYSTEM MESSAGES":string)
            n985 = case shown="True" "Clear All Messages" {
              selector: "Clear All Messages" -> [_ w1277]
              frame False {
              }
              frame True {
                n986 = call "Monta_Mensagem.vi"("Zerar"=w1277) -> ()  [unwired: 2 in]
              }
            }
            n987 = local read "alarm Time"() -> (w1256:timestamp)
            n988 = Get Date/Time In Seconds() -> (seconds since 1Jan1904=w1255:timestamp)
            n989 = Greater?(x=w1255, y=w1256) -> (0:w1257:bool)
            n990 = case shown="True" w1257 {
              frame False {
              }
              frame True {
                n991 = local read "Flag Alarm"() -> (w1270:bool)
                n992 = case shown="True" w1270 {
                  selector: w1270 -> [_ w1273]
                  frame False {
                  }
                  frame True {
                    n993 = Not(x=w1273) -> (.not. x?=w1272:bool)
                    n994 = property on="Mensage Alarme" class="Str"("Visible"=FALSE) -> ()  [unwired: 2 in, 2 out]
                    n995 = local write "Flag Alarm"(w1272) -> ()
                  }
                }
              }
            }
          }
          frame #13 {
            w1300 = u16 3 items=["Alarme", "Atencao", "Erro", "Ocupado", "Protecao", "Embreagem", "Tracking", "Var. Track", "Rápido", "Ligeiro", "Médio", "Lento", "Em movimento", ""] ("NomeStatus")
            w1301 = u16 3 items=["Alarme", "Atencao", "Erro", "Ocupado", "Protecao", "Embreagem", "Tracking", "Var. Track", "Rápido", "Ligeiro", "Médio", "Lento", "Em movimento", ""] ("NomeStatus")
            # "PROCESSO AQUISIÇÃO"
            n996 = global read "Global_Telescopio.vi" "Correção Aquis"() -> (w1296:bool)
            n997 = call "Bit Status AH.vi"("NomeStatus"=w1301) -> ("StatBit"=w1298:bool)
            n998 = call "Bit Status DEC.vi"("NomeStatus"=w1300) -> ("StatBit"=w1299:bool)
            n999 = Not Or(1:w1299, 2:w1298) -> (0:w1297:bool)
            n1000 = Compound Arithmetic op=AND(w1296, w1297) -> (w1302:bool)
            n1001 = case shown="True" w1302 {
              frame False {
              }
              frame True {
                # "Reseta Flag do movimento de\n offset do Sist de Aquisição"
                n1002 = global read "Global_Telescopio.vi" "CorrecaoMin"() -> (w1308:dbl)
                n1003 = global read "Global_Telescopio.vi" "aquis_asc"() -> (w1307:dbl)
                n1004 = global read "Global_Telescopio.vi" "aquis_dec"() -> (w1310:dbl)
                n1005 = Absolute Value(x=w1310) -> (abs(x)=w1306:dbl)
                n1006 = global read "Global_Telescopio.vi" "CorrecaoMin"() -> (w1311:dbl)
                n1007 = global write "Global_Telescopio.vi" "Correção Aquis"(FALSE ("Correção Aquis")) -> ()
                n1008 = Absolute Value(x=w1307) -> (abs(x)=w1305:dbl)
                n1009 = Greater?(x=w1306, y=w1311) -> (0:w1312:bool)
                n1010 = Greater?(x=w1305, y=w1308) -> (0:w1309:bool)
                n1011 = case shown="True" w1309 {
                  tunnel: w1307 -> [_ w1313]
                  frame False {
                  }
                  frame True {
                    w1315 = u16 1 items=["ZERO", "AH", "DEC", "TUBO", "CUP"] ("Controlador")
                    # "PROCESSO MOVE TELESCÓPIO"
                    n1012 = call "Conversao Ms to Hora texto.vi"("TRUE=HORA\nFALSE=GRAU"=TRUE ("TRUE=HORA\nFALSE=GRAU"), "PrecDEC"=w1313) -> ("Hora/Graus Texto Decimal"=w1318:string)
                    n1013 = call "Monta Comando.vi"("Set Point"=w1318, "Comando"="MOVER_REL", "Dispositivo"="EIXO" ("Comando"), "Controlador"=w1315) -> ()  [unwired: 3 in, 3 out]
                  }
                }
                n1014 = case shown="True" w1312 {
                  tunnel: w1310 -> [_ w1319]
                  frame False {
                  }
                  frame True {
                    w1321 = u16 2 items=["ZERO", "AH", "DEC", "TUBO", "CUP"] ("Controlador")
                    # "PROCESSO MOVE TELESCÓPIO"
                    n1015 = call "Conversao Ms to Hora texto.vi"("TRUE=HORA\nFALSE=GRAU"=FALSE ("TRUE=HORA\nFALSE=GRAU"), "PrecDEC"=w1319) -> ("Hora/Graus Texto Decimal"=w1324:string)
                    n1016 = call "Monta Comando.vi"("Set Point"=w1324, "Comando"="MOVER_REL", "Dispositivo"="EIXO" ("Comando"), "Controlador"=w1321) -> ()  [unwired: 3 in, 3 out]
                  }
                }
                n1017 = global write "Global_Telescopio.vi" "AQ Offset Mov"(TRUE ("AQ Offset Mov")) -> ()
              }
            }
          }
          frame #14 {
            w1337 = "\r\n"
            # "MUDANÇA 10/8/2010 \nIncluídos:\n- Nome do instrumento\n- RA do telescópio"
            # "OBS: O Arquivo é inicialmente apagado para \nEvitar que fique corrompido!"
            # "Escreve arquivo com Dados para o Uso da Página do PDA"
            n1018 = global read "Global_Telescopio.vi" "Lista Instrumentos"() -> (w1339:string[])
            n1019 = global read "Global_Telescopio.vi" "Sideral Time"() -> (w1329:dbl)
            n1020 = global read "Global_Telescopio.vi" "PosAH"() -> (w1330:dbl)
            n1021 = global read "Global_Telescopio.vi" "Instrum"() -> (w1338:u16)
            n1022 = local read "DOMO_ENC"() -> (w1351:string)
            n1023 = local read "Sideral time"() -> (w1358:string)
            n1024 = local read "CUP_STAT"() -> (w1347:string)
            n1025 = local read "AH_STAT"() -> (w1349:string)
            n1026 = local read "AH_ENC"() -> (w1353:string)
            n1027 = local read "UT"() -> (w1357:string)
            n1028 = Subtract(x=w1329, y=w1330) -> (x-y=w1334:dbl)
            n1029 = Add(x=6.283185307179586, y=w1334) -> (x+y=w1333:dbl)
            n1030 = Less Than 0?(x=w1334) -> (x < 0?=w1331:bool)
            n1031 = call "Retira_tudo_depois_da_virgula.vi"("Entrada"=w1358) -> ("Saída"=w1355:string)
            n1032 = local read "TUBO_STAT"() -> (w1346:string)
            n1033 = Format Date/Time String(time format string (%c)="%H:%M:%S") -> (date/time string=w1341:string)  [unwired: 2 in]
            n1034 = local read "FOCO_ENC"() -> (w1350:string)
            n1035 = local read "DEC_STAT"() -> (w1348:string)
            n1036 = local read "DEC_ENC"() -> (w1352:string)
            n1037 = Select(t=w1333, s=w1331, f=w1334) -> (s? t:f=w1335:dbl)
            n1038 = Index Array(array=w1339, index=w1338) -> (element=w1340:string)
            n1039 = Format Date/Time String(time format string (%c)="%d/%m/%Y") -> (date/time string=w1342:string)  [unwired: 2 in]
            n1040 = call "Retira_tudo_depois_da_virgula.vi"("Entrada"=w1357) -> ("Saída"=w1354:string)
            n1041 = call <vilib>:"Trim Whitespace.vi"("string"=w1355) -> ("trimmed string"=w1345:string)  [unwired: 1 in]
            n1042 = call "rad_hms.vi"("TRUE=HORA\nFALSE=GRAU"=TRUE, "Radiano"=w1335) -> ("Hora/Graus Texto Decimal"=w1328:string)  [unwired: 3 in]
            n1043 = String To Path(string="C:\\TCS\\ARQUIVOS\\DadosTCSPD.txt") -> (path=w1359:path)
            n1044 = Concatenate Strings(w1342, w1337, w1341, w1337, w1354, w1337, w1345, w1337, w1353, w1337, w1352, w1337, w1351, w1337, w1350, w1337, w1349, w1337, w1348, w1337, w1347, w1337, w1346, w1337, w1340, w1337, w1328, w1337) -> (w1361:string)
            n1045 = case shown="True" "Case Constant\n(See Context Help) 2" {
              tunnel: [w1370 w1373] -> w1360
              tunnel: w1359 -> [w1370 w1372]
              frame False {
              }
              frame True {
                n1046 = Delete(path (use dialog)=w1372) -> (deleted path=w1373:path, error out=→"error out":errorcluster)  [unwired: 4 in, 1 out]
              }
            }
            n1047 = call <vilib>:"Open_Create_Replace File.vi"("function (open:0)"=T7."open or create", "file path"=w1360) -> ("error out"=w1365:errorcluster, "refnum"=w1368:refnum<file>)  [unwired: 6 in, 2 out]
            n1048 = Set File Position(refnum=w1368, from (0:start)=enum16{"start", "end", "current"}."start" ("pos mode (0:2)"), error in=w1365) -> (refnum out=w1327:refnum<file>, error out=w1326:errorcluster)  [unwired: 1 in]
            n1049 = Write to Binary File(file (use dialog)=w1327, data=w1361, error in=w1326, 5:FALSE ("prepend array or string size? (T)")) -> (refnum out=w1367:refnum<file>, error out=w1366:errorcluster)  [unwired: 2 in, 1 out]
            n1050 = Close File(refnum=w1367, error in=w1366) -> (error out=w1369:errorcluster)  [unwired: 1 out]
            n1051 = call <vilib>:"Simple Error Handler.vi"("error in (no error)"=w1369) -> ()  [unwired: 4 in, 5 out]
          }
          frame #15 {
            # "Página do PDA"
            # "http://192.168.1.1:1080/pdaWeb/"
            # "TRATAMENTO DO PDA"
            n1052 = stacked-sequence {
              frame #0 {
                # "MUDANÇA  3/9/2010 \nIncluído case abaixo e código de seu estado TRUE para apagar eventuais comandos do PDA enviados antes do TCSPD rodar."
                n1053 = First Call?() -> (First Call?: T/F=w1374:bool)
                n1054 = case shown="True" w1374 {
                  frame False {
                    # "MUDANÇA  4/9/2010 \nSubstituída a VI \"New Read PPC\" pela \"Trata PDA\" a qual evita que o telescópio seja apontado para regiões proibidas (inclinação excessiva)."
                    # "lê e interpreta o arquivo ppc.txt"
                    n1055 = call "Trata PDA.vi"() -> ()  [unwired: 2 in]
                  }
                  frame True {
                    n1056 = call "Find ppctxt.vi"() -> ("Existe ppc.txt?"=w1376:bool, "ppc.txt Path"=w1375:path)  [unwired: 1 in]
                    n1057 = case shown="True" w1376 {
                      tunnel: w1375 -> [_ w1377]
                      frame False {
                      }
                      frame True {
                        # "limpa o arquivo ppc.txt"
                        n1058 = call "Wipe file.vi"("ppc path"=w1377) -> ()  [unwired: 2 out]
                      }
                    }
                  }
                }
              }
              frame #1 {
                n1059 = case shown="False" "Case Constant\n(See Context Help) 3" {
                  frame False {
                  }
                  frame True {
                    # "MUDANÇA:\nÉ necesário \nsubstituir as variáveis simuladas pelas do Sistema"
                    # "Simula os dados sendo alterados pela\nmovimentação do sistema"
                    n1060 = call "Data Table.vi"() -> ()  [unwired: 1 in]
                  }
                }
              }
              frame #2 {
                n1061 = case shown="True" "Case Constant\n(See Context Help) 4" {
                  frame False {
                  }
                  frame True {
                    # "Lê o arquivo padrão para o equip/o\nselecionado pelo PDA e grava o\narquivo ppcDisplay.htm adequado"
                    n1062 = call "Update Frame.vi"() -> ("Timeout"=w1380:u32)  [unwired: 2 in, 3 out]
                    n1063 = Wait Until Next ms Multiple(millisecond multiple=w1380) -> ()  [unwired: 1 out]
                  }
                }
              }
            }
          }
        }
        n1064 = global read "Global_Telescopio.vi" "Flag-Rotator"() -> (w73:bool)
        n1065 = case shown="True" w73 {
          frame False {
          }
